vi "CreatePrivateEvents.vi"(8 "error in (no error)":errorcluster, 11 "SignalReceiver":refnum<class "SignalReceiver.lvclass">) -> (0 "error out":errorcluster, 3 "SignalReceiver out":refnum<class "SignalReceiver.lvclass">)   [LabVIEW 2020, in "ECU_Diagnose.lvlib" / "SignalReceiver.lvclass"]
doc: "JKI State Machine Objects (SMO) 1.1.0.20\nJKI - JKI\nCopyright (c) 2016, JKI"
uses:
  SignalReceiver.lvclass
  SignalReceiver.lvclass/SignalReceiver.ctl
  Typedefs/AsyncMethodInputs--Cluster.ctl
  Typedefs/PrivateEvents--SignalReceiver.Start_Stop.ctl
  <vilib>/JKI/JKI SMO/SMO/SMO.lvclass
panel:
  # "For instructions on how to use the JKI State Machine Objects, examples and video tutorials, visit:\nhttp://jki.net/state-machine-objects/\n\nJKI State Machine Objects™\nhttp://jki.net/state-machine-objects/\nCopyright (C) 2005-2015, JKI <info@jki.net>\nALL RIGHTS RESERVED"
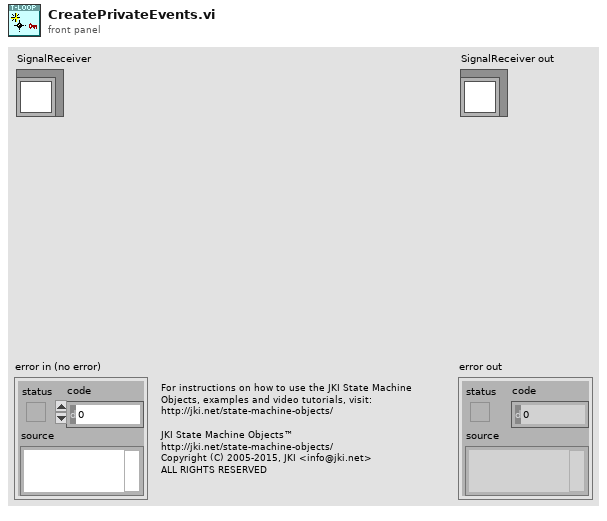
[diagram p1: front panel]
types:
  T1 = typedef "ECU_Diagnose.lvlib/SignalReceiver.lvclass/PrivateData--Ref.ctl" = refnum<data-value>
  T2 = typedef "ECU_Diagnose.lvlib/SignalReceiver.lvclass/PrivateEvents--SignalReceiver.Start_Stop.ctl" = bool
  T3 = typedef "ECU_Diagnose.lvlib/SignalReceiver.lvclass/AsyncMethodInputs--Cluster.ctl" = cluster{"Data":dbl}
  T4 = typedef "ECU_Diagnose.lvlib/SignalReceiver.lvclass/PrivateData--Cluster.ctl" = cluster{"Public Events":T5, "Private Events":T6, "SignalArrySelect":T7, "SignalDataReciArry":T8}
  T5 = typedef "ECU_Diagnose.lvlib/SignalReceiver.lvclass/PublicEvents--Cluster.ctl" = cluster{"Setpoint Changed":refnum<user-event>, "Value Changed":refnum<user-event>}
  T6 = typedef "ECU_Diagnose.lvlib/SignalReceiver.lvclass/PrivateEvents--Cluster.ctl" = cluster{"AsyncMethod":refnum<user-event>, "Start_Stop":refnum<user-event>}
  T7 = typedef "ECU_Diagnose.lvlib/SignalReceiver.lvclass/SignalArrySelecte.ctl" = cluster{"Port_No.":refnum<k21>, "XNET Signal":refnum<k21>[]}
  T8 = typedef "ECU_Diagnose.lvlib/SignalReceiver.lvclass/SignalDataArry.ctl" = cluster{"SignalDataReceiveArry":dbl[][], "Update":bool}
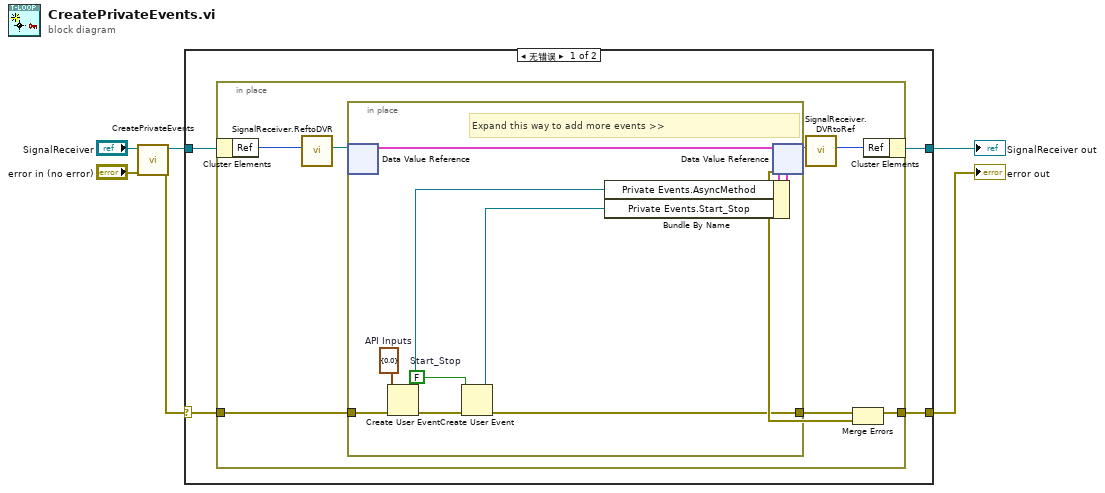
[diagram p0: block diagram]
diagram:
  n1 = call-parent "CreatePrivateEvents.vi"("error in (no error)"="error in (no error)", "SMO"="SignalReceiver") -> ("error out"=w4:errorcluster, "SMO out"=w2:refnum<class "SignalReceiver.lvclass">)  [unwired: 8 in]
  n2 = case shown="无错误" w4 {
    selector: w4 -> [w8 w29]
    tunnel: [w7 w29] -> w3
    tunnel: [w9 w28] -> w1
    tunnel: w2 -> [w10 w28]
    frame No Error {
      n3 = in-place {
        in-place-border: w8 -> [w18]
        in-place-border: [w15] -> w7
        n4 = in-place-cluster #1(w10) -> ("Ref"=w14:u32)
        n5 = call "SignalReceiver.ReftoDVR.vi"("Ref"=w14) -> ("Ref"=w13:T1)  [unwired: 10 in]
        n6 = in-place {
          in-place-border: w18 -> [w25]
          in-place-border: [w21] -> w17
          w20 = T2 FALSE  # Start_Stop
          w22 = T3 {"Data"=0.0}  # API Inputs
          # "Expand this way to add more events >>"
          n7 = in-place-dvr #2(w13) -> (w24:T4)  [unwired: 1 out]
          n8 = Create User Event(user event datatype=w22, error in=w25) -> (user event=w23:refnum<user-event>, error out=w26:errorcluster)
          n9 = Create User Event(user event datatype=w20, error in=w26) -> (user event=w19:refnum<user-event>, error out=w21:errorcluster)
          n10 = Bundle By Name(cluster=w24, "Private Events.AsyncMethod"=w23, "Private Events.Start_Stop"=w19) -> (w27:T4)
          n11 = in-place-dvr #2(w27) -> (w12:T1, w16:errorcluster)
        }
        n12 = call "SignalReceiver.DVRtoRef.vi"("Ref"=w12) -> ("Ref"=w11:u32)  [unwired: 10 in]
        n13 = Merge Errors(w17, w16) -> (w15:errorcluster)
        n14 = in-place-cluster #1("Ref"=w11) -> (w9:refnum<class "SignalReceiver.lvclass">)
      }
    }
    frame Error {
    }
  }
  "error out" <- w3
  "SignalReceiver out" <- w1
